vi "test Add Find Remove Analog Replay.vi"(8 "error in (no error)":errorcluster, 11 "TestCase in":refnum<class "Scripting API Test Case.lvclass">) -> (0 "error out":errorcluster, 3 "TestCase out":refnum<class "Scripting API Test Case.lvclass">)   [LabVIEW 2015, in "Scripting API Test Case.lvclass"]
uses:
  Scripting API Test Case.lvclass
  Scripting API/Custom Device/Engine Simulation Toolkit Custom Device Settings.ctl
  Scripting API/Bitfile/Bitfile.ctl
  Scripting API/Analog Replay/Analog Replay Settings.ctl
  Scripting API/Analog Replay/Analog Replay Data Options.ctl
  System Explorer/FPGA Mem Size.ctl
  System Explorer/Position Reference.ctl
  System Explorer/Data Replay Data Selection Method.ctl
  NationalInstruments.VeriStand.SystemDefinitionAPI
  <userlib>/_OpenG.lib/file/file.llb/Append Path to Root if Relative - Scalar__ogtk.vi
  <vilib>/addons/_JKI Toolkits/VI Tester/TestCase.llb/TestCase.lvclass
  niveristand-custom-device-testing-tools/VeriStandTestUtilities/VeriStandTestUtilities.lvlib
  Scripting API/Engine Simulation Toolkit Scripting API.lvlib
  System Explorer/Engine Simulation Toolkit System Explorer.lvlib
panel:
  in  "Save?":bool
  out "Output Filename":string
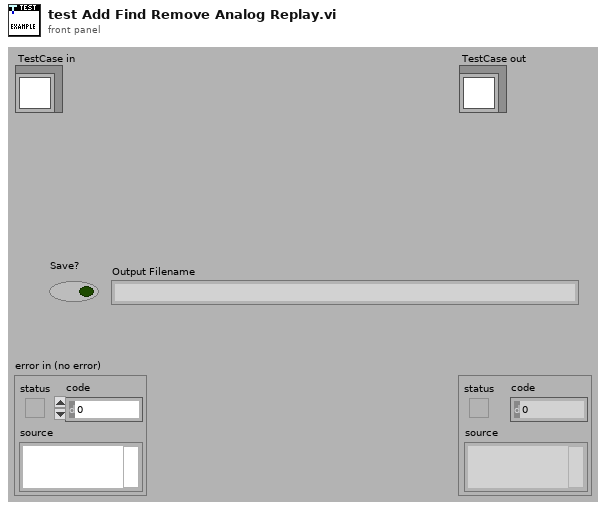
[diagram p1: front panel]
types:
  T1 = typedef "Engine Simulation Toolkit Scripting API.lvlib/Analog Replay Data Options.ctl" = cluster{"Selected File":path, "Group":string, "Channel":string, "DataPlugin":string, "ReverseData":bool, "FPGA memory size":T2, "CycleAngle?":T3, "Data Selection Method":T4, "File start offset":i32, "Samples":i32, "Missing teeth location (degrees)":dbl}
  T2 = typedef "Engine Simulation Toolkit System Explorer.lvlib/FPGA Mem Size.ctl" = enum16{"65,536", "32,768", "16,384", "8,192", "4,096", "2,048", "1,024"}
  T3 = typedef "Engine Simulation Toolkit System Explorer.lvlib/Position Reference.ctl" = enum16{"Crank angle", "Cycle angle"}
  T4 = typedef "Engine Simulation Toolkit System Explorer.lvlib/Data Replay Data Selection Method.ctl" = enum32{"Manual", "AutoVRCrank"}
  T5 = typedef "Engine Simulation Toolkit Scripting API.lvlib/Bitfile.ctl" = cluster{"RIO Device Address":string, "Bitfile Path":path}
  T6 = typedef "Engine Simulation Toolkit Scripting API.lvlib/Engine Simulation Toolkit Custom Device Settings.ctl" = cluster{"Name":string, "Execution priority":enum16{"Low", "Medium", "High"}, "Rate decimation":i32, "CPU":i32}
  T7 = typedef "Engine Simulation Toolkit Scripting API.lvlib/Analog Replay Settings.ctl" = cluster{"Name":string, "RIO Device Address":string, "DAC bipolar range (V)":dbl, "Voltage below min speed":dbl, "Min speed (RPM)":dbl, "Voltage at min speed":dbl, "Max speed (RPM)":dbl, "Voltage at max speed":dbl, "ReverseNegate":bool, "VOverride":bool}
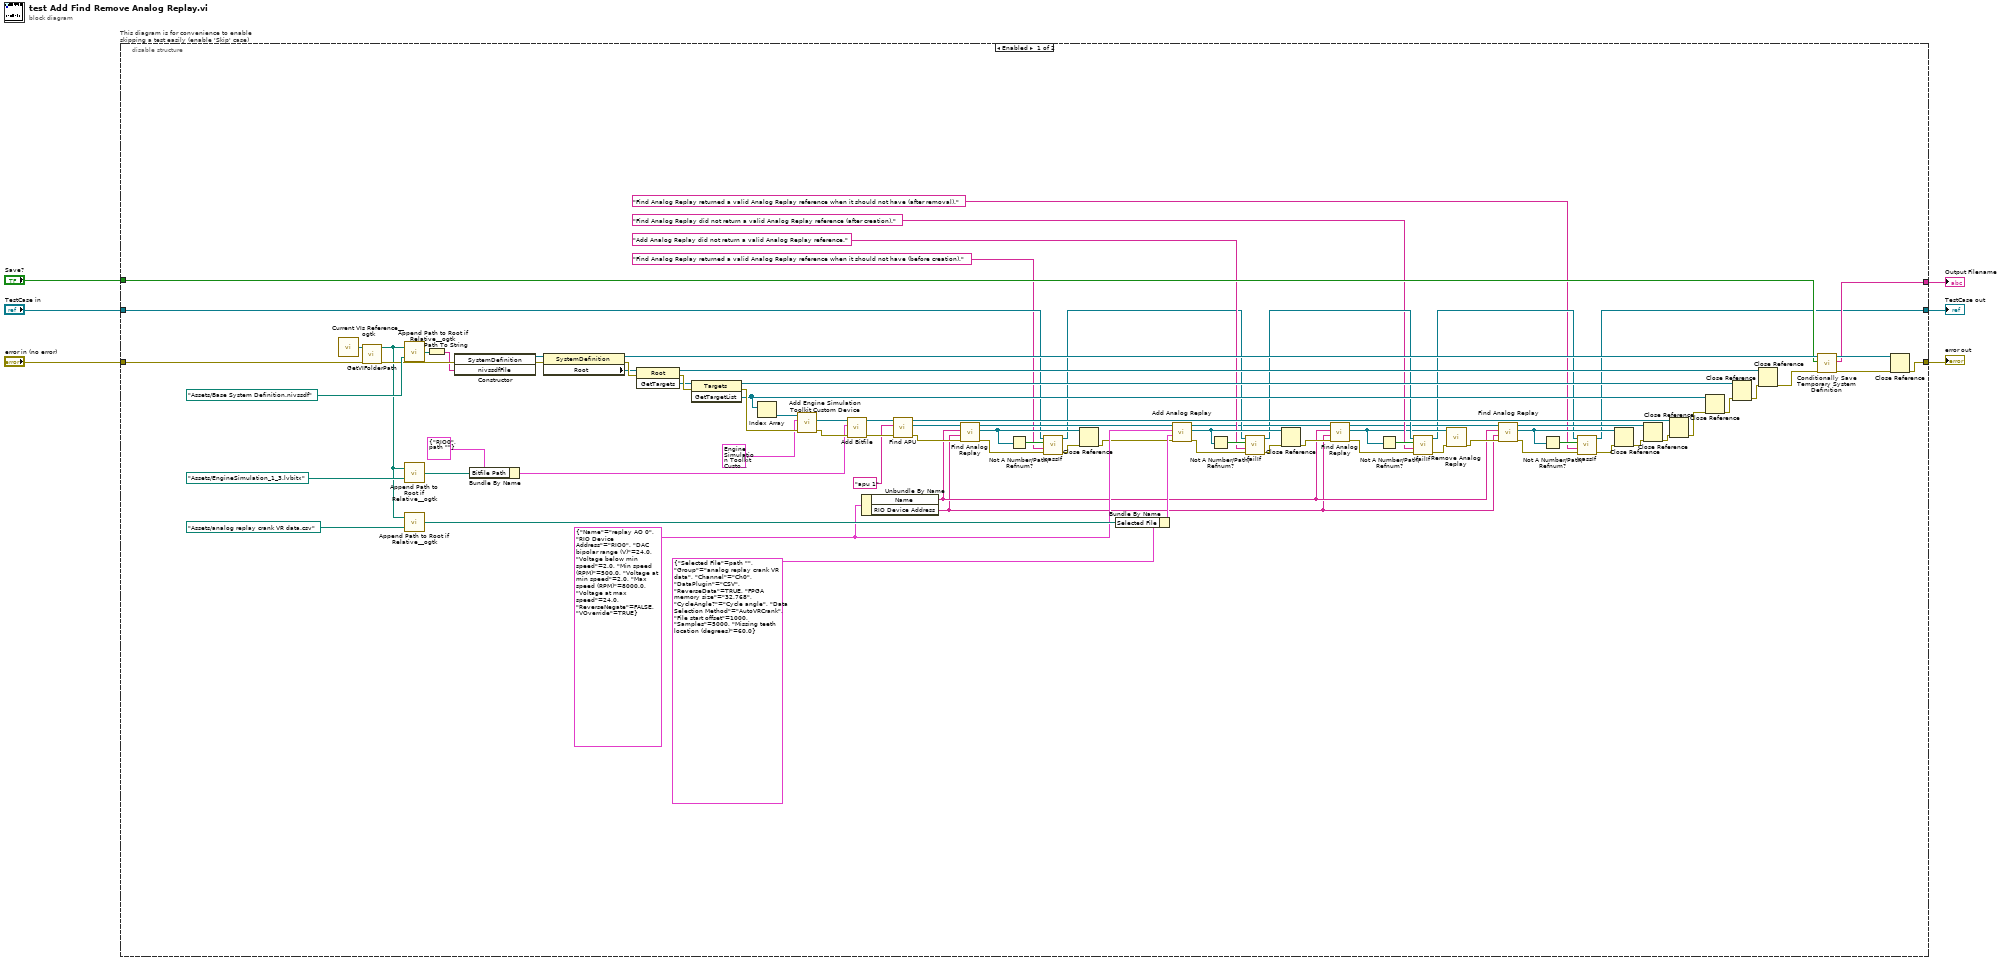
[diagram p0: block diagram]
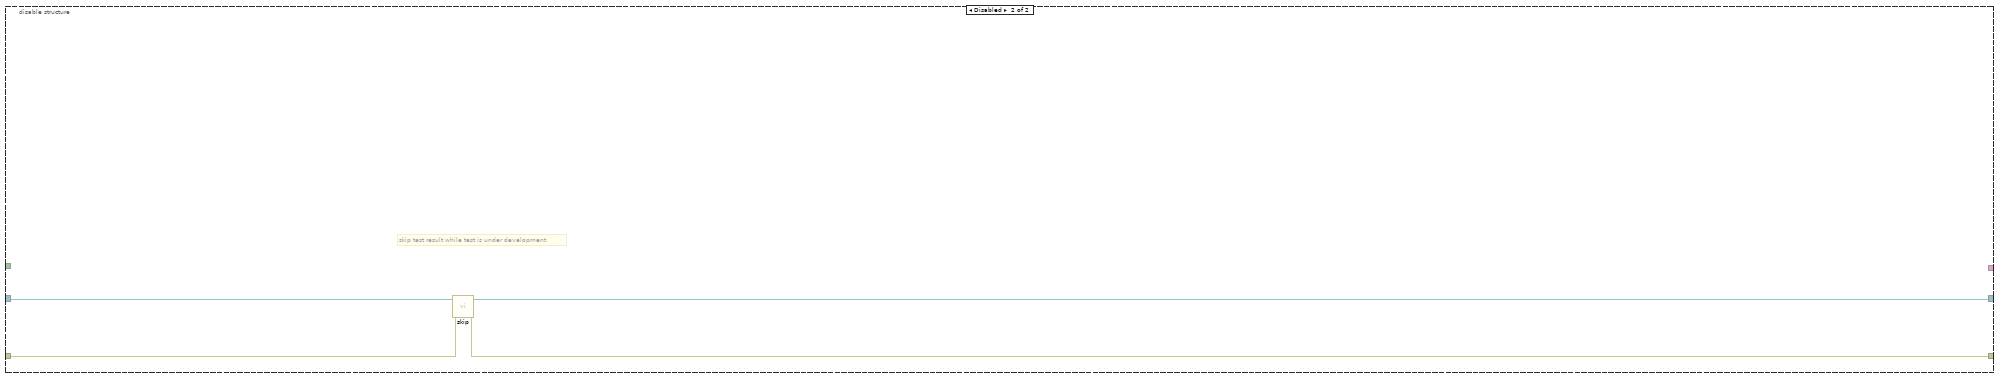
[diagram p2: hidden frame]
diagram:
  n1 = disable-structure "This diagram is for convenience to enable skipping a test easily (enable 'Skip' case)" shown="Enabled" {
    disable-tunnel: "TestCase in" -> [w31 w92]
    disable-tunnel: [w9 w90] -> w3
    disable-tunnel: [w80 w91] -> w5
    disable-tunnel: "error in (no error)" -> [w87 w89]
    disable-tunnel: [w63 _] -> w2
    disable-tunnel: "Save?" -> [w62 _]
    frame Enabled {
      w39 = T7 {"Name"="replay AO 0", "RIO Device Address"="RIO0", "DAC bipolar range (V)"=24.0, "Voltage below min speed"=2.0, "Min speed (RPM)"=500.0, "Voltage at min speed"=2.0, "Max speed (RPM)"=8000.0, "Voltage at max speed"=24.0, "ReverseNegate"=FALSE, "VOverride"=TRUE} ("Analog Replay Settings")
      n2 = call <userlib>:"Current VIs Reference__ogtk.vi"() -> ("Current VI's reference"=w88:refnum<vi>)  [unwired: 5 in]
      n3 = call "GetVIFolderPath.vi"("error in (no error)"=w87, "VI Reference in"=w88) -> ("error out"=w84:errorcluster, "VI Folder Path out"=w47:path)  [unwired: 8 in]
      n4 = call-poly <userlib>:"Append Path to Root if Relative__ogtk.vi"("Absolute or Relative Path"=path "Assets/Base System Definition.nivssdf", "Root Path"=w47) -> ("Absolute or Appended Path"=w85:path)
      n5 = call-poly <userlib>:"Append Path to Root if Relative__ogtk.vi"("Absolute or Relative Path"=path "Assets/EngineSimulation_1_3.lvbitx", "Root Path"=w47) -> ("Absolute or Appended Path"=w55:path)
      n6 = call-poly <userlib>:"Append Path to Root if Relative__ogtk.vi"("Absolute or Relative Path"=path "Assets/analog replay crank VR data.csv", "Root Path"=w47) -> ("Absolute or Appended Path"=w46:path)
      n7 = Path To String(path=w85) -> (string=w82:string)
      n8 = constructor class="SystemDefinition"(error in=w84, "nivssdfFile"=w82) -> (reference out=w81:refnum<k24>, error out=w83:errorcluster)  [unwired: 2 in, 2 out]
      n9 = Bundle By Name(cluster=T5 {"RIO Device Address"="RIO0", "Bitfile Path"=path ""} ("Engine Simulation Toolkit Bitfile"), "Bitfile Path"=w55) -> (w56:T5)
      n10 = property class="SystemDefinition"(reference=w81, error in=w83) -> (reference out=w65:refnum<k24>, error out=w78:errorcluster, "Root"=w77:refnum<k24>)
      n11 = invoke class="Root" method="GetTargets"(reference=w77, error in=w78) -> (reference out=w79:refnum<k24>, error out=w74:errorcluster, "GetTargets"=w73:refnum<k24>)  [unwired: 1 in]
      n12 = invoke class="Targets" method="GetTargetList"(reference=w73, error in=w74) -> (reference out=w75:refnum<k24>, error out=w70:errorcluster, "GetTargetList"=w69:refnum<k24>[])  [unwired: 1 in]
      n13 = Index Array(array=w69) -> (element=w71:refnum<k24>)  [unwired: 1 in]
      n14 = call "Add Engine Simulation Toolkit Custom Device.vi"("error in (no error)"=w70, "Settings"=T6 {"Name"="Engine Simulation Toolkit Custom Device", "Execution priority"=enum."Medium", "Rate decimation"=1, "CPU"=-2} ("Engine Simulation Toolkit Custom Device Settings"), "Target in"=w71) -> ("error out"=w59:errorcluster, "EST Custom Device"=w61:refnum<k24>)  [unwired: 6 in, 1 out]
      n15 = call "Add Bitfile.vi"("error in (no error)"=w59, "Engine Simulation Toolkit Bitfile"=w56, "EST Custom Device in"=w61) -> ("error out"=w53:errorcluster, "EST Custom Device out"=w54:refnum<k24>)  [unwired: 7 in]
      n16 = Unbundle By Name(w39) -> ("Name"=w17:string, "RIO Device Address"=w16:string)
      n17 = call "Find APU.vi"("error in (no error)"=w53, "Name"="apu 1", "EST Custom Device in"=w54) -> ("error out"=w36:errorcluster, "APU"=w38:refnum<k24>, "EST Custom Device out"=w52:refnum<k24>)  [unwired: 6 in]
      n18 = call "Find Analog Replay.vi"("error in (no error)"=w36, "RIO Device Address"=w16, "Name"=w17, "APU in"=w38) -> ("error out"=w32:errorcluster, "Analog Replay"=w34:refnum<k24>, "APU out"=w37:refnum<k24>)  [unwired: 5 in]
      n19 = Not A Number/Path/Refnum?(number/path/refnum=w34) -> (NaN/Path/Refnum?=w35:bool)
      n20 = call-dynamic "passIf.vi"("error in (no error)"=w32, "message (\"\")"="Find Analog Replay returned a valid Analog Replay reference when it should not have (before creation)." ("message (\"\")"), "pass"=w35, "TestCase in"=w31) -> ("error out"=w33:errorcluster, "TestCase out"=w30:refnum<class "Scripting API Test Case.lvclass">)  [unwired: 6 in]
      n21 = Close Reference(reference=w34, error in (no error)=w33) -> (error out=w28:errorcluster)
      n22 = Bundle By Name(cluster=T1 {"Selected File"=path "", "Group"="analog replay crank VR data", "Channel"="Ch0", "DataPlugin"="CSV", "ReverseData"=TRUE, "FPGA memory size"=enum."32,768", "CycleAngle?"=enum."Cycle angle", "Data Selection Method"=enum."AutoVRCrank", "File start offset"=1000, "Samples"=5000, "Missing teeth location (degrees)"=60.0} ("Analog Replay Data Options"), "Selected File"=w46) -> (w48:T1)
      n23 = call "Add Analog Replay.vi"("error in (no error)"=w28, "Analog Replay Data Options"=w48, "Analog Replay Settings"=w39, "APU in"=w37) -> ("error out"=w43:errorcluster, "Analog Replay"=w42:refnum<k24>, "APU out"=w25:refnum<k24>)  [unwired: 5 in]
      n24 = Not A Number/Path/Refnum?(number/path/refnum=w42) -> (NaN/Path/Refnum?=w44:bool)
      n25 = call-dynamic "failIf.vi"("error in (no error)"=w43, "message (\"\")"="Add Analog Replay did not return a valid Analog Replay reference." ("message (\"\")"), "fail"=w44, "TestCase in"=w30) -> ("error out"=w40:errorcluster, "TestCase out"=w23:refnum<class "Scripting API Test Case.lvclass">)  [unwired: 6 in]
      n26 = Close Reference(reference=w42, error in (no error)=w40) -> (error out=w24:errorcluster)
      n27 = call "Find Analog Replay.vi"("error in (no error)"=w24, "RIO Device Address"=w16, "Name"=w17, "APU in"=w25) -> ("error out"=w26:errorcluster, "Analog Replay"=w21:refnum<k24>, "APU out"=w19:refnum<k24>)  [unwired: 5 in]
      n28 = Not A Number/Path/Refnum?(number/path/refnum=w21) -> (NaN/Path/Refnum?=w27:bool)
      n29 = call-dynamic "failIf.vi"("error in (no error)"=w26, "message (\"\")"="Find Analog Replay did not return a valid Analog Replay reference (after creation)." ("message (\"\")"), "fail"=w27, "TestCase in"=w23) -> ("error out"=w20:errorcluster, "TestCase out"=w10:refnum<class "Scripting API Test Case.lvclass">)  [unwired: 6 in]
      n30 = call "Remove Analog Replay.vi"("error in (no error)"=w20, "Analog Replay"=w21) -> ("error out"=w18:errorcluster)  [unwired: 9 in]
      n31 = call "Find Analog Replay.vi"("error in (no error)"=w18, "RIO Device Address"=w16, "Name"=w17, "APU in"=w19) -> ("error out"=w7:errorcluster, "Analog Replay"=w14:refnum<k24>, "APU out"=w12:refnum<k24>)  [unwired: 5 in]
      n32 = Not A Number/Path/Refnum?(number/path/refnum=w14) -> (NaN/Path/Refnum?=w15:bool)
      n33 = call-dynamic "passIf.vi"("error in (no error)"=w7, "message (\"\")"="Find Analog Replay returned a valid Analog Replay reference when it should not have (after removal)." ("message (\"\")"), "pass"=w15, "TestCase in"=w10) -> ("error out"=w13:errorcluster, "TestCase out"=w9:refnum<class "Scripting API Test Case.lvclass">)  [unwired: 6 in]
      n34 = Close Reference(reference=w14, error in (no error)=w13) -> (error out=w11:errorcluster)
      n35 = Close Reference(reference=w12, error in (no error)=w11) -> (error out=w50:errorcluster)
      n36 = Close Reference(reference=w52, error in (no error)=w50) -> (error out=w68:errorcluster)
      n37 = Close Reference(reference=w69, error in (no error)=w68) -> (error out=w72:errorcluster)
      n38 = Close Reference(reference=w75, error in (no error)=w72) -> (error out=w76:errorcluster)
      n39 = Close Reference(reference=w79, error in (no error)=w76) -> (error out=w64:errorcluster)
      n40 = call "Conditionally Save Temporary System Definition.vi"("error in (no error)"=w64, "Save?"=w62, ".NET Refnum in"=w65) -> ("error out"=w67:errorcluster, "filename"=w63:string, ".NET Refnum out"=w66:refnum<k24>)  [unwired: 6 in]
      n41 = Close Reference(reference=w66, error in (no error)=w67) -> (error out=w80:errorcluster)
    }
    frame Disabled {
      # "skip test result while test is under development"
      n42 = call <vilib>:"skip.vi"("error in (no error)"=w89, "TestCase in"=w92) -> ("error out"=w91:errorcluster, "TestCase out"=w90:refnum<class "Scripting API Test Case.lvclass">)  [unwired: 8 in]
    }
  }
  "error out" <- w5
  "TestCase out" <- w3
  "Output Filename" <- w2
